vi "single_channel_demod.vi"() -> ()   [LabVIEW 2014]
uses:
  <vilib>/rvi/FXPMathLib/FxpAtan2/subVIs/nifxpmath_Atan2_SimConfig.ctl
  <vilib>/rvi/FXPMathLib/FxpAtan2/simVIs/DllFxpAtan2Temp_sub.vi
  <vilib>/rvi/FXPMathLib/FxpAtan2/XNode/nifxpmath_Atan2.xnode
  <vilib>/rvi/Analysis/measure/butterworth/XNode/niFpgaButterworthFilter.xnode
panel:
  in  "lpf_config":T1={"scaled coefficients"=[-859855294, 1909791330, 5951447], "channel index"=0}
  out "amp_filt_out":fxp<+/-,36,18> format="%.23g"
  out "counter_out":u8
  out "phi_out":fxp<+/-,16,2>
  out "n_out":i16
  in  "counter_in":u8
  in  "sig":i16
  in  "phase_in":fxp<+/-,17,3>=1.0
  in  "n_in":i16
  in  "discont_pos":fxp<+/-,17,3>=1.0
  in  "discont_neg":fxp<+/-,3,2>=-1.0
  out "amp_out":fxp<+,34,16> format="%.23g"
  in  "Counter Offset":u8
  out "phi_full_filt_out":fxp<+/-,36,18> format="%.20g"
  in  "use lpf?":bool
  in  "c3_mult":i16=1
  in  "c3_delay_mult":i16=-1
  in  "c2_mult":i16=-1
  in  "c2_delay_mult":i16=-1
  in  "c1_mult":i16=-1
  in  "c1_delay_mult":i16=1
  in  "c0_mult":i16=1
  in  "c0_delay_mult":i16=1
  in  "Reset Phi":bool
  out "phi_full_out":fxp<+/-,32,18>=2.0 format="%.20g"
  out "n":i16
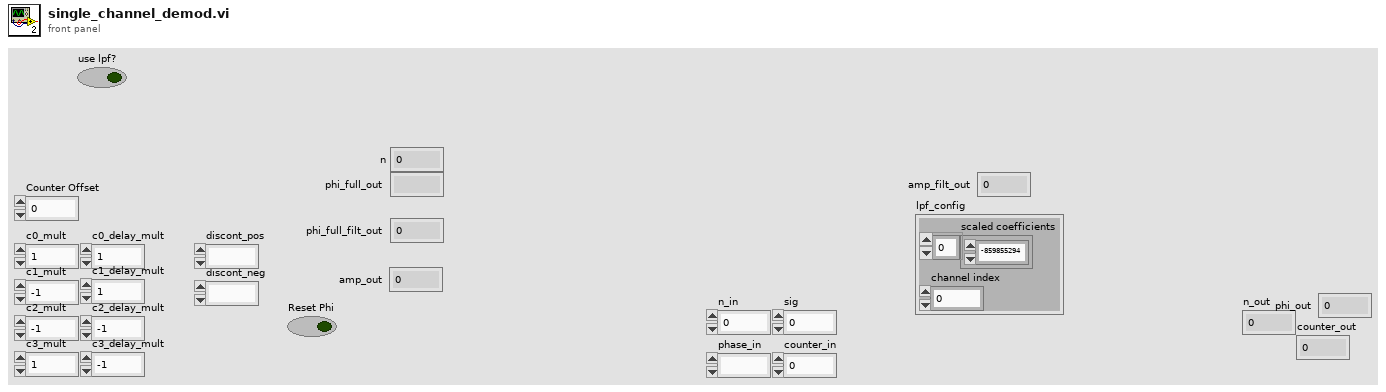
[diagram p1: front panel]
types:
  T1 = cluster{"scaled coefficients":i32[], "channel index":u16}
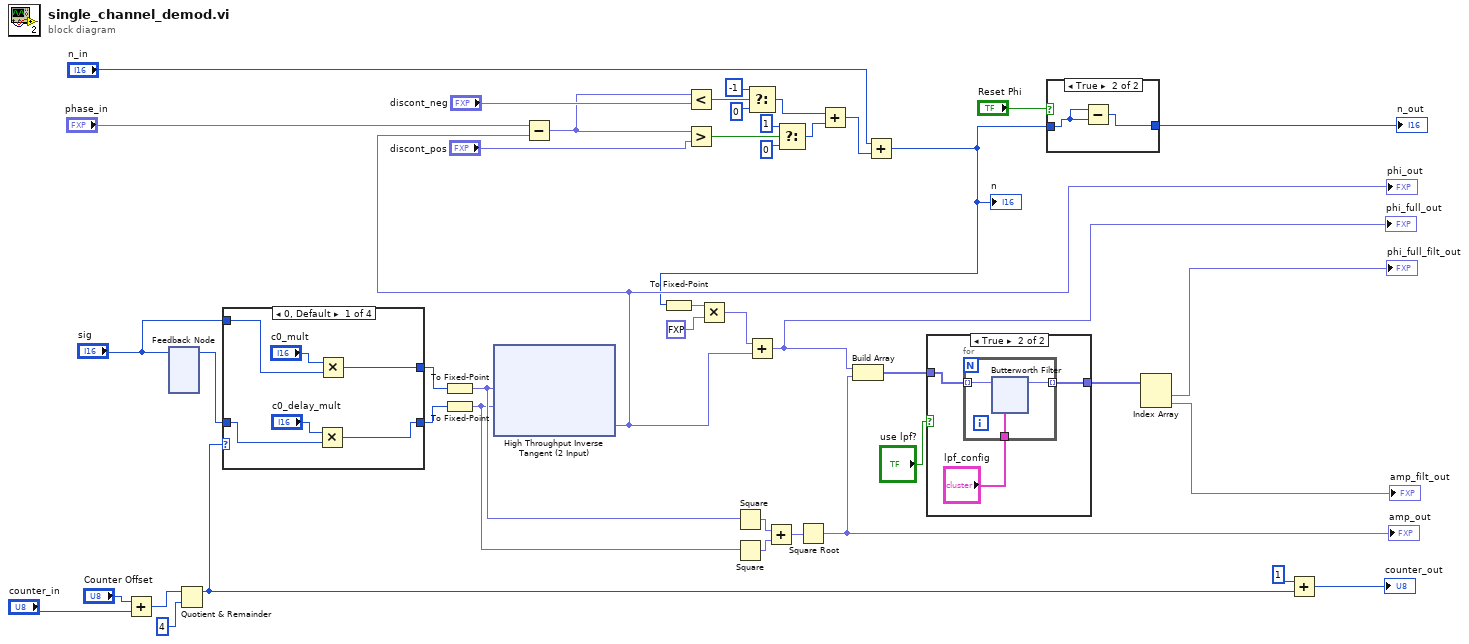
[diagram p0: block diagram]
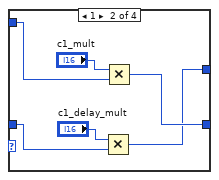
[diagram p3: hidden frame]
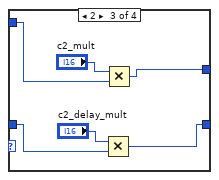
[diagram p4: hidden frame]
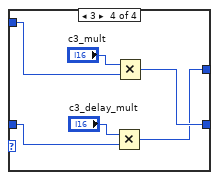
[diagram p5: hidden frame]
diagram:
  n1 = Add(x="Counter Offset", y="counter_in") -> (x+y=w36:u8)
  n2 = feedback #1() -> (w41:i16)  [unwired: 1 in]
  n3 = feedback-in #1("sig") -> ()
  n4 = Quotient & Remainder(x=w36, y=u8 4) -> (x-y*floor(x/y)=w35:u8)  [unwired: 1 out]
  n5 = case shown="0, Default" w35 {
    tunnel: "sig" -> [w48 w54 w60 w66]
    tunnel: w41 -> [w47 w52 w58 w65]
    tunnel: [w46 w53 w57 w64] -> w39
    tunnel: [w45 w51 w59 w63] -> w40
    frame 0, Default {
      n6 = Multiply(x="c0_delay_mult", y=w47) -> (x*y=w46:i16)
      n7 = Multiply(x="c0_mult", y=w48) -> (x*y=w45:i16)
    }
    frame 1 {
      n8 = Multiply(x="c1_delay_mult", y=w52) -> (x*y=w51:i16)
      n9 = Multiply(x="c1_mult", y=w54) -> (x*y=w53:i16)
    }
    frame 2 {
      n10 = Multiply(x="c2_delay_mult", y=w58) -> (x*y=w57:i16)
      n11 = Multiply(x="c2_mult", y=w60) -> (x*y=w59:i16)
    }
    frame 3 {
      n12 = Multiply(x="c3_delay_mult", y=w65) -> (x*y=w63:i16)
      n13 = Multiply(x="c3_mult", y=w66) -> (x*y=w64:i16)
    }
  }
  n14 = To Fixed-Point(number=w40) -> (fixed-point=w34:fxp<+/-,16,16>)  [unwired: 1 in]
  n15 = To Fixed-Point(number=w39) -> (fixed-point=w33:fxp<+/-,16,16>)  [unwired: 1 in]
  n16 = xnode "High Throughput Inverse Tangent (2 Input)"("y"=w34, "x"=w33) -> ("atan2(y,x) (pi)"=w12:fxp<+/-,16,2>)
  "phi_out" <- w12
  n17 = Subtract(x="phase_in", y=w12) -> (x-y=w18:fxp<+/-,18,4>)
  n18 = Less?(x=w18, y="discont_neg") -> (x < y?=w20:bool)
  n19 = Greater?(x=w18, y="discont_pos") -> (0:w24:bool)
  n20 = Square(x=w34) -> (x^2=w28:fxp<+,31,31>)
  n21 = Square(x=w33) -> (x^2=w29:fxp<+,31,31>)
  n22 = Select(t=i16 -1, s=w20, f=i16 0) -> (s? t:f=w25:i16)
  n23 = Add(x=w28, y=w29) -> (x+y=w30:fxp<+,32,32>)
  n24 = Select(t=i16 1, s=w24, f=i16 0) -> (s? t:f=w26:i16)
  n25 = Square Root(x=w30) -> (sqrt(x)=w8:fxp<+,34,16>)
  "amp_out" <- w8
  n26 = Add(x=w25, y=w26) -> (x+y=w27:i16)
  n27 = Add(x="n_in", y=w27) -> (x+y=w5:i16)
  "n" <- w5
  n28 = To Fixed-Point(number=w5) -> (fixed-point=w6:fxp<+/-,16,16>)  [unwired: 1 in]
  n29 = Multiply(x=w6, y=fxp<+,1,2> 2.0) -> (x*y=w1:fxp<+/-,16,17>)
  n30 = Add(x=w1, y=w12) -> (x+y=w9:fxp<+/-,32,18>)
  "phi_full_out" <- w9
  n31 = Build Array(w9, w8) -> (w10:fxp<+/-,36,18>[])
  n32 = case shown="True" "use lpf?" {
    tunnel: w10 -> [w69 w72]
    tunnel: [w69 w71] -> w4
    frame False {
    }
    frame True {
      n33 = for {
        tunnel: w72 -> [w75] mode=indexing
        tunnel: [w74] -> w71 mode=indexing
        tunnel: "lpf_config" -> [w73]
        n34 = xnode "Butterworth Filter"("input data"=w75, "configuration"=w73) -> ("output data"=w74:fxp<+/-,16,18>)  [unwired: 1 in, 1 out]
      }
    }
  }
  n35 = case shown="True" "Reset Phi" {
    tunnel: w5 -> [w85 w86]
    tunnel: [w85 w87] -> w13
    frame False {
    }
    frame True {
      n36 = Subtract(x=w86, y=w86) -> (x-y=w87:i16)
    }
  }
  "n_out" <- w13
  n37 = Index Array(array=w4) -> (element #1=→"phi_full_filt_out":fxp<+/-,36,18>, element #2=→"amp_filt_out":fxp<+/-,36,18>)  [unwired: 2 in]
  n38 = Add(x=u8 1, y=w35) -> (x+y=→"counter_out":u8)
